vi "Write freq.vi"(8 "error in (no error)":errorcluster, 10 "freq":dbl, 11 "MultiUsrp in":refnum<class "MultiUsrp.lvclass">) -> (0 "error out":errorcluster, 3 "MultiUsrp out":refnum<class "MultiUsrp.lvclass">)   [LabVIEW 2023, in "uhd.lvlib" / "MultiUsrp.lvclass"]
uses:
  <userlib>/uhd/MultiUsrp/MultiUsrp.lvclass
  <userlib>/uhd/MultiUsrp/MultiUsrp.lvclass/MultiUsrp.ctl
  <userlib>/uhd/uhd.lvlib
  <userlib>/uhd/usrp session.ctl
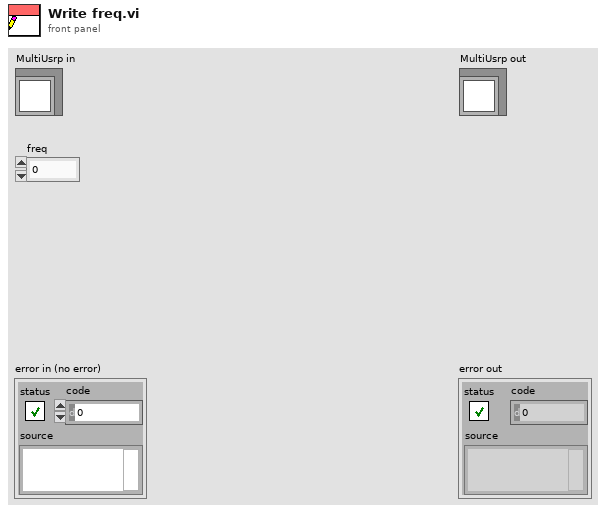
[diagram p1: front panel]
types:
  T1 = typedef "usrp session.ctl" = cluster{"h":u64, "Enum":enum16{"usrp handle"}}
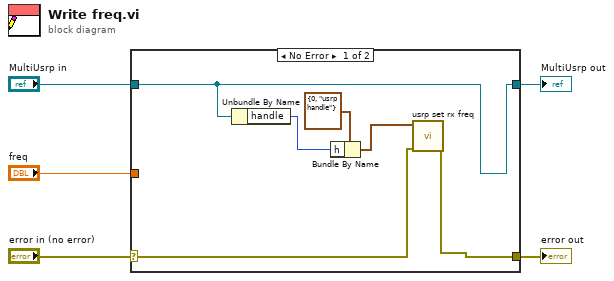
[diagram p0: block diagram]
diagram:
  n1 = case shown="No Error" "error in (no error)" {
    selector: "error in (no error)" -> [w8 w12]
    tunnel: [w7 w12] -> w4
    tunnel: [w6 w13] -> w2
    tunnel: "MultiUsrp in" -> [w6 w13]
    tunnel: "freq" -> [_ _]
    frame No Error {
      n2 = Unbundle By Name(w6) -> ("handle"=w10:u64)
      n3 = Bundle By Name(cluster=T1 {"h"=0, "Enum"=enum."usrp handle"} ("h"), "h"=w10) -> (w9:T1)
      n4 = call <userlib>:"usrp set rx freq.vi"("error in (no error)"=w8, "h"=w9) -> ("error out"=w7:errorcluster)  [unwired: 4 in, 5 out]
    }
    frame Error {
    }
  }
  "error out" <- w4
  "MultiUsrp out" <- w2
